vi "Save To File (SubVI).vi"(8 "error in (no error)":errorcluster, 9 "array type (2D Dbl)":dbl[](array[numeric]), 10 "Save data":bool, 11 "file path (dialog if empty)":path) -> (0 "error out":errorcluster)   [LabVIEW 2021]
uses:
  <vilib>/Utility/file.llb/Write Delimited Spreadsheet (DBL).vi
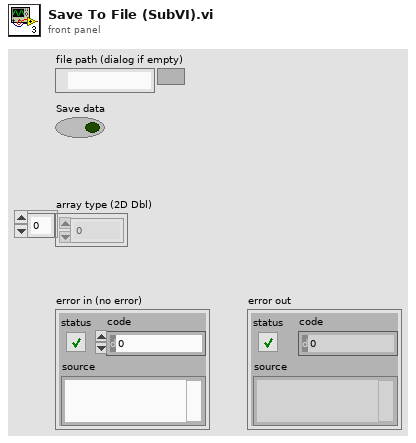
[diagram p1: front panel]
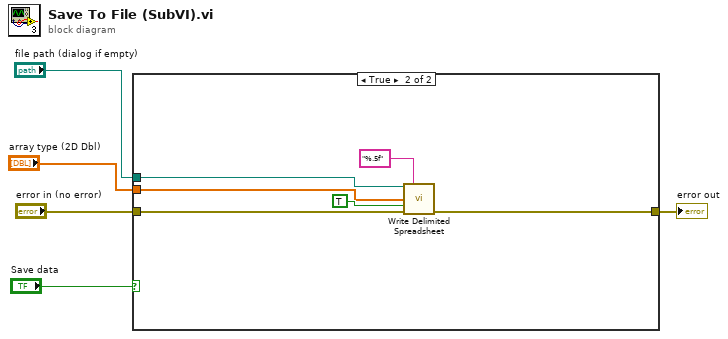
[diagram p0: block diagram]
diagram:
  n1 = case shown="True" "Save data" {
    tunnel: "file path (dialog if empty)" -> [_ w12]
    tunnel: "array type (2D Dbl)" -> [_ w9]
    tunnel: "error in (no error)" -> [w6 w8]
    tunnel: [w6 w7] -> w4
    frame False {
    }
    frame True {
      n2 = call-poly <vilib>:"Write Delimited Spreadsheet.vi"("file path (dialog if empty)"=w12, "format (%.3f)"="%.5f", "1D data"=w9, "append to file? (new file:F)"=TRUE, "error in (no error)"=w8) -> ("error out"=w7:errorcluster)  [unwired: 9 in, 1 out]
    }
  }
  "error out" <- w4
